vi "Spin Coat LbL Krizak SMS.vi"() -> ()   [LabVIEW 2018]
uses:
  <vilib>/ErrorRing/Error Ring.xnode
panel:
  in  "Units in 5":string(combo)="mh"
  in  "Set rate in 5":dbl=400.0
  in  "dia (mm) in 5":dbl=24.0 min=0.1 max=50.0 step=0.1
  in  "Units in 4":string(combo)="mh"
  in  "Set rate in 4":dbl=400.0
  in  "dia (mm) in 4":dbl=24.0 min=0.1 max=50.0 step=0.1
  in  "Units in 3":string(combo)="mh"
  in  "Set rate in 3":dbl=400.0
  in  "dia (mm) in 3":dbl=33.0 min=0.1 max=50.0 step=0.1
  in  "Units in 2":string(combo)="mh"
  in  "Set rate in 2":dbl=400.0
  in  "dia (mm) in 2":dbl=24.0 min=0.1 max=50.0 step=0.1
  out "Invalid Recipient":string
  in  "SMS Updates":bool=TRUE
  in  "Carrier":string(combo)="@tmomail.net"
  in  "Phone number":string="2816302191"
  out "Complete Indicator":bool caption="Start Button"
  in  "Activate Pump 5":bool
  out "Stopped 5":bool
  in  "Address in 5":string(combo)="0"
  in  "Target Vol (mL) 5":dbl=0.9
  out "Dispensed (mL) 5":dbl
  out "Success 5":bool
  out "Spin Coater":bool
  out "Pumps":bool
  out "Stopped 4":bool
  in  "Address in 4":string(combo)="3"
  in  "Target Vol (mL) 4":dbl=0.9
  out "Dispensed (mL) 4":dbl
  out "Success 4":bool
  out "Stopped 3":bool
  in  "Address in 3":string(combo)="4"
  in  "Target Vol (mL) 3":dbl=0.9
  out "Dispensed (mL) 3":dbl
  out "Success 3":bool
  out "Stopped 2":bool
  in  "Address in 2":string(combo)="1"
  in  "Target Vol (mL) 2":dbl=0.9
  out "Dispensed (mL) 2":dbl
  out "Success 2":bool
  out "Stopped 1":bool
  out "Pumps Reads":string
  out "Pump Commands":string
  out "Pump Reads Length":string
  in  "Address in 1":string(combo)="2"
  in  "Target Vol (mL) 1":dbl=0.9
  in  "Units in":string(combo)="mh"
  in  "Direction in":bool=TRUE
  in  "Set rate in":dbl=400.0
  in  "dia (mm) in":dbl=24.0 min=0.1 max=50.0 step=0.1
  in  "Pumps Serial Port":refnum<visa-resource-name>="COM1"
  out "Pump Operating":i32
  out "Layer #":i32=1
  out "String  After Match":string
  out "String  Before Match":string
  out "String  Match":string
  out "Spin Coater Stopped":bool
  in  "VISA resource name":refnum<visa-resource-name>="COM4" caption="Spin Coater Serial Port"
  out "Match 3":u8
  out "Match 2":u8
  out "Match 4":u8
  out "Match 5":u8
  out "Match 1":u8
  out "Match #":i32
  out "Spin Coater Reads":string
  out "error out":errorcluster
  in  "Stop All Button":bool caption="Start Button"
  out "Dispensed (mL) 1":dbl
  out "Success 1":bool
  in  "Number of Layers":i32=30
  # "Warning: This program must be started prior to starting the spin coater"
  # "Set pump Baud rate to 19200"
  # "Note: Spin Coater must be programmed independently for the correct number of cycles at a proper spin speed."
  # "Pump 1"
  # "Pump 2"
  # "Pump 5"
  # "Pump 3"
  # "Pump 4"
  # "Monomer 1"
  # "Rinse"
  # "Monomer 2"
  # "Rinse"
  # "Graphene"
  # "Diagnostics Panel"
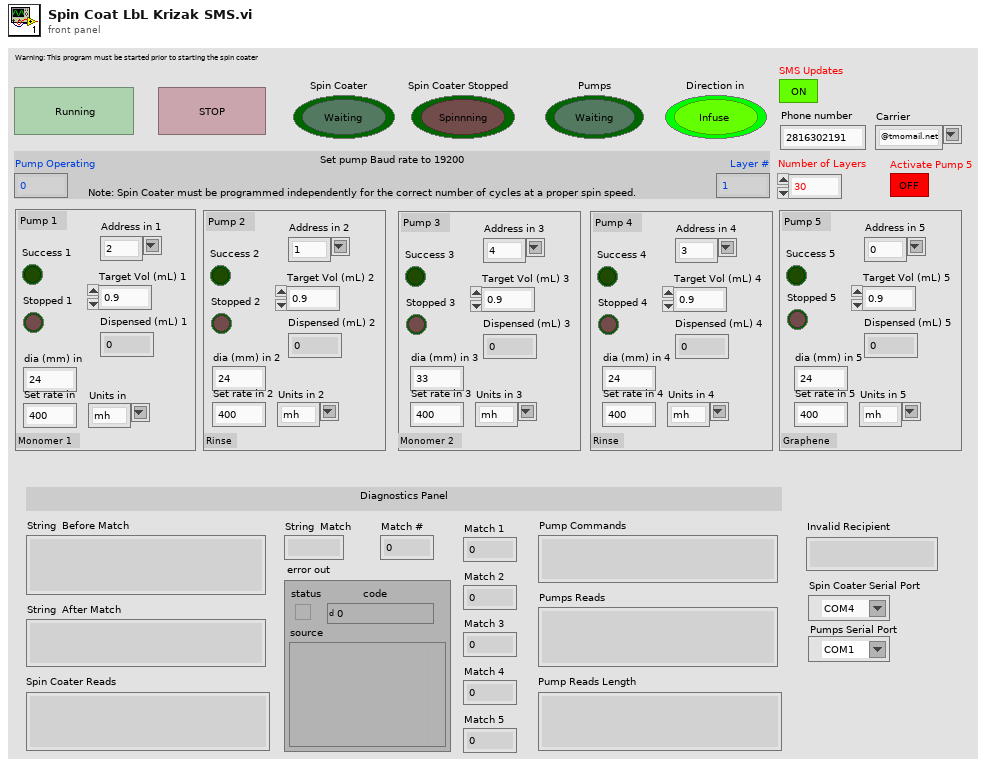
[diagram p1: front panel]
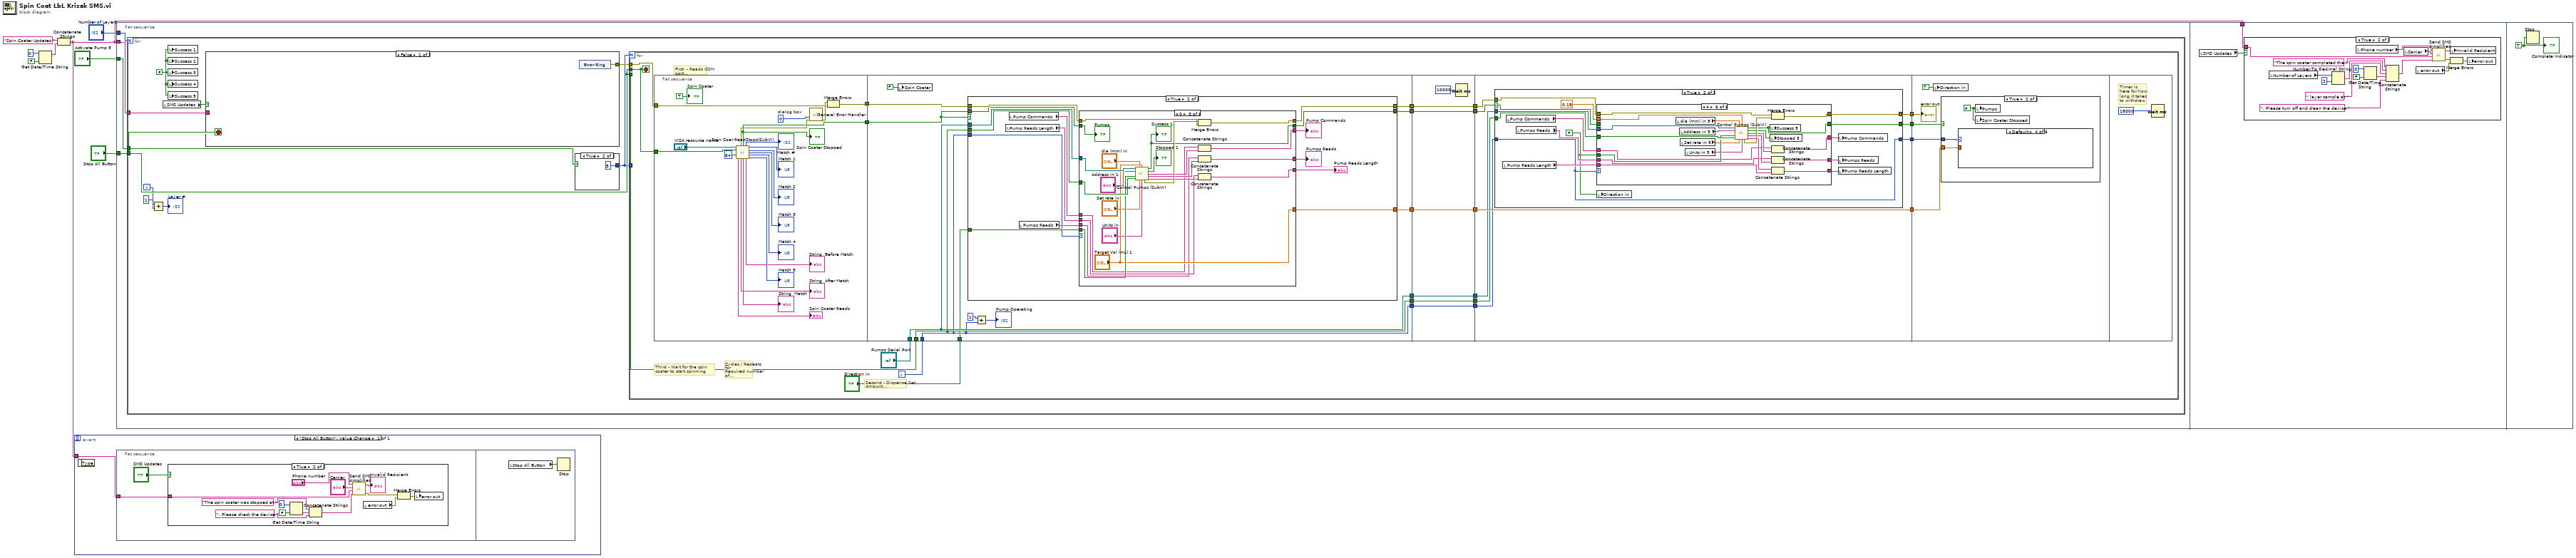
[diagram p0: block diagram]
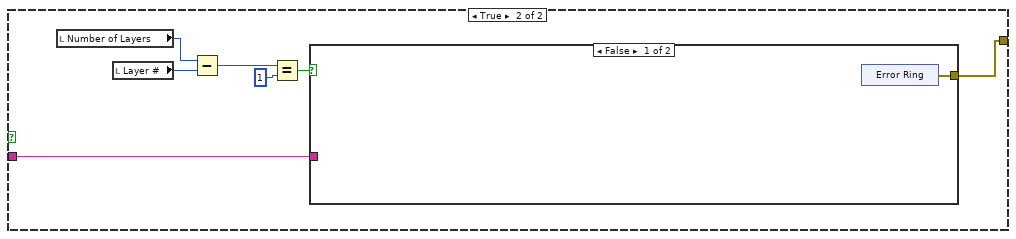
[diagram p2: hidden frame]
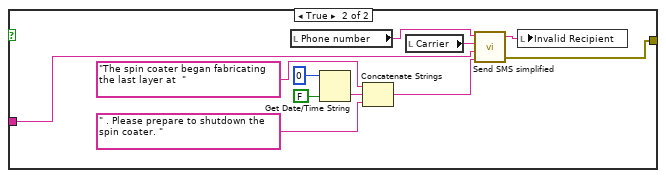
[diagram p3: hidden frame]
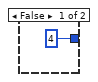
[diagram p4: hidden frame]
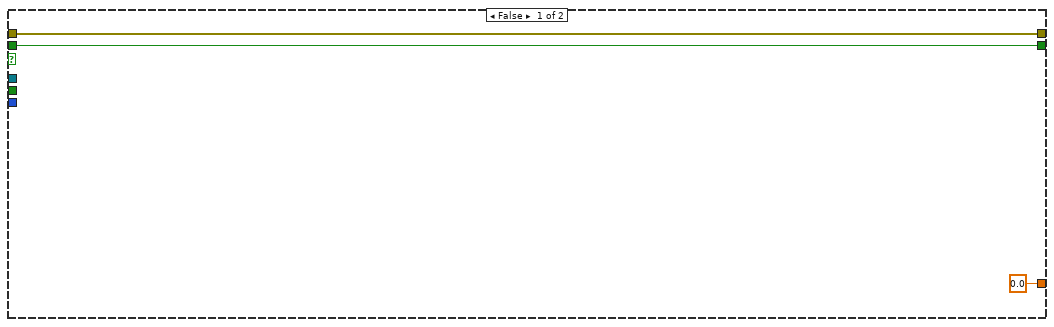
[diagram p5: hidden frame]
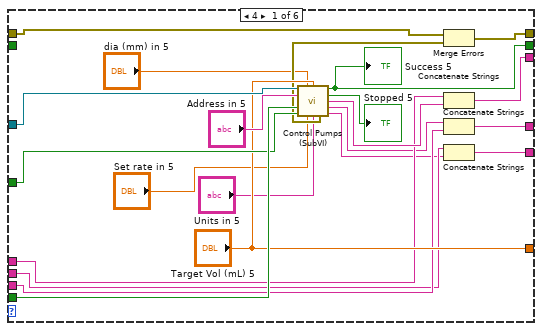
[diagram p6: hidden frame]
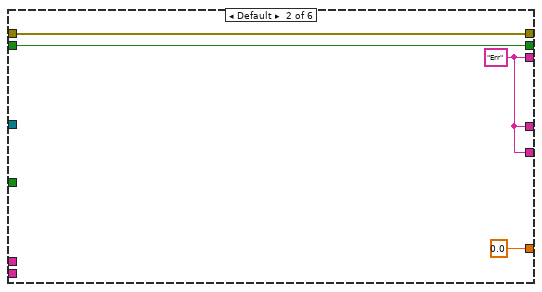
[diagram p7: hidden frame]
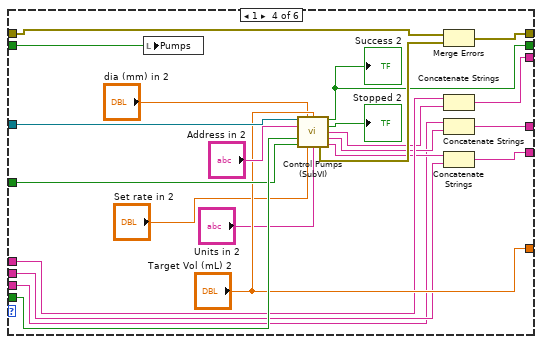
[diagram p8: hidden frame]
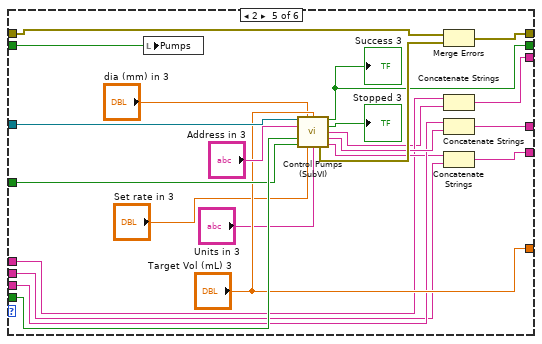
[diagram p9: hidden frame]
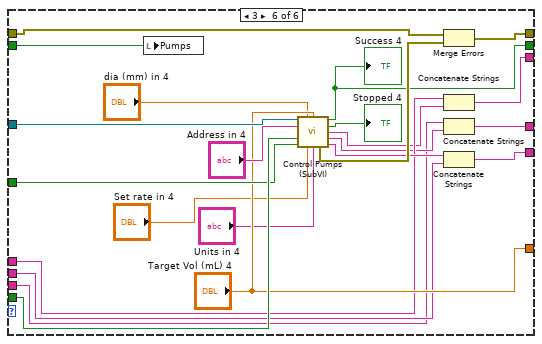
[diagram p10: hidden frame]
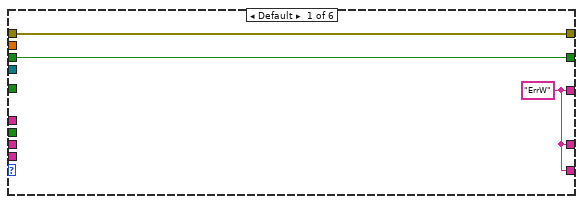
[diagram p12: hidden frame]
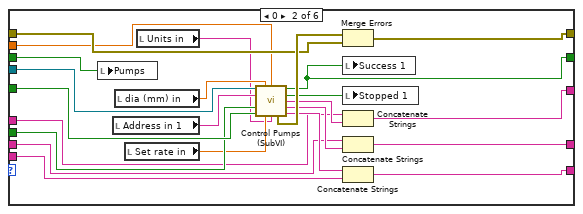
[diagram p13: hidden frame]
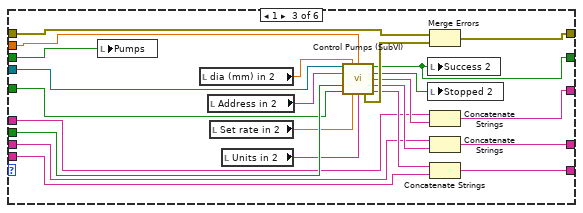
[diagram p14: hidden frame]
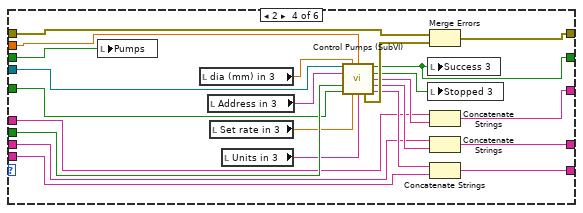
[diagram p15: hidden frame]
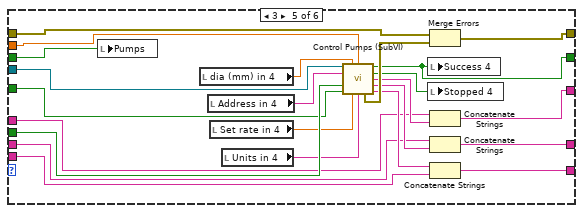
[diagram p16: hidden frame]
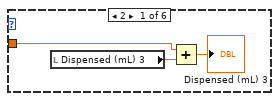
[diagram p18: hidden frame]
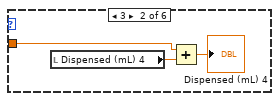
[diagram p19: hidden frame]
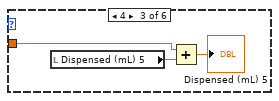
[diagram p20: hidden frame]
diagram:
  n1 = Get Date/Time String(date format (0)=i8 0 ("Number of pumps"), want seconds? (F)=FALSE) -> (date string=w2:string)  [unwired: 1 in, 1 out]
  n2 = Concatenate Strings("Spin Coater Updates ", w2) -> (w1:string)
  n3 = event shown="[0] \"Stop All Button\": Value Change" {
    selector: _ -> [_]
    dyn-events: _ -> [_]
    timeout: _ -> [_]
    tunnel: w1 -> [w9]
    event "Stop All Button": Value Change {
      n4 = event-data() -> ()  [unwired: 1 in, 1 out]
      n5 = flat-sequence {
        tunnel: w9 -> [w10]
        frame #0 {
          n6 = case shown="True" "SMS Updates" {
            tunnel: w10 -> [_ w23]
            frame False {
              n7 = xnode "Error Ring"() -> ()  [unwired: 1 out]
            }
            frame True {
              n8 = Get Date/Time String(date format (0)=i8 0 ("Number of pumps"), want seconds? (F)=FALSE) -> (time string=w19:string)  [unwired: 1 in, 1 out]
              n9 = Concatenate Strings("The spin coater was stopped at ", w19, ". Please check the device.") -> (w18:string)
              n10 = call "Send SMS simplified.vi"("Message"=w18, "Subject"=w23, "Carrier"="Carrier", "Phone number"="Phone number") -> ("Error Out"=w14:errorcluster, "Invalid Recipients"=→"Invalid Recipient":string)  [unwired: 1 in]
              n11 = local read "error out"() -> (w15:errorcluster)
              n12 = Merge Errors(w14, w15) -> (w13:errorcluster)
              n13 = local write "error out"(w13) -> ()
            }
          }
        }
        frame #1 {
          n14 = local read "Stop All Button"() -> (w26:bool)
          n15 = Stop(stop? (T)=w26) -> ()
        }
      }
    }
  }
  n16 = flat-sequence {
    tunnel: "Stop All Button" -> [w30]
    tunnel: "Activate Pump 5" -> [w29]
    tunnel: "Number of Layers" -> [w28]
    tunnel: w1 -> [w27]
    tunnel: w1 -> [w432]
    frame #0 {
      n17 = for {
        N: w28 -> [_]
        tunnel: w30 -> [w40]
        tunnel: w29 -> [w39]
        tunnel: w27 -> [w32]
        i -> [w37]
        stop <- w40 stop-if-true
        w34 = FALSE
        n18 = Add(x=1, y=w37) -> (x+y=→"Layer #":i32)
        n19 = local read "SMS Updates"() -> (w33:bool)
        n20 = local write "Success 1"(w34) -> ()
        n21 = local write "Success 2"(w34) -> ()
        n22 = local write "Success 3"(w34) -> ()
        n23 = local write "Success 4"(w34) -> ()
        n24 = local write "Success 5"(w34) -> ()
        n25 = case shown="False" w33 {
          tunnel: w32 -> [_ w44]
          tunnel: [w41 w43] -> w31
          frame False {
            n26 = xnode "Error Ring"() -> ("error out"=w41:errorcluster)
          }
          frame True {
            n27 = local read "Number of Layers"() -> (w49:i32)
            n28 = local read "Layer #"() -> (w48:i32)
            n29 = Subtract(x=w49, y=w48) -> (x-y=w46:i32)
            n30 = Equal?(x=w46, y=1) -> (x = y?=w47:bool)
            n31 = case shown="False" w47 {
              tunnel: w44 -> [_ w62]
              tunnel: [w50 w58] -> w43
              frame False {
                n32 = xnode "Error Ring"() -> ("error out"=w50:errorcluster)
              }
              frame True {
                n33 = local read "Phone number"() -> (w61:string)
                n34 = Get Date/Time String(date format (0)=i8 0 ("Number of pumps"), want seconds? (F)=FALSE) -> (time string=w55:string)  [unwired: 1 in, 1 out]
                n35 = Concatenate Strings("The spin coater began fabricating the last layer at  ", w55, " . Please prepare to shutdown the spin coater. ") -> (w53:string)
                n36 = local read "Carrier"() -> (w60:string)
                n37 = call "Send SMS simplified.vi"("Message"=w53, "Subject"=w62, "Carrier"=w60, "Phone number"=w61) -> ("Error Out"=w58:errorcluster, "Invalid Recipients"=w59:string)  [unwired: 1 in]
                n38 = local write "Invalid Recipient"(w59) -> ()
              }
            }
          }
        }
        n39 = case shown="True" w39 {
          tunnel: [4 ("Number of pumps") 5 ("Number of pumps")] -> w35
          frame False {
          }
          frame True {
          }
        }
        n40 = for {
          N: w35 -> [_]
          tunnel: w40 -> [w88]
          tunnel: w40 -> [w85]
          tunnel: w35 -> [_]
          tunnel: w31 -> [w65]
          i -> [w66]
          stop <- w88 stop-if-true
          # "Cycles / Repeats for \nRequired number of \nmonomers and\nlayers"
          # "Second - Dispense Set Amount\nfrom a given pump"
          # "Third - Wait for the spin \ncoater to start spinning"
          # "First  - Reads COM port\n   until spin coater stops"
          n41 = flat-sequence {
            tunnel: [w90] -> w87
            tunnel: [w105] -> w86
            tunnel: w88 -> [w107]
            tunnel: w65 -> [w89]
            tunnel: w87 -> [w120]
            tunnel: w86 -> [w115]
            tunnel: w66 -> [w110]
            tunnel: w85 -> [w112]
            tunnel: "Pumps Serial Port" -> [w114]
            tunnel: "Direction in" -> [w113]
            tunnel: [w119] -> w78
            tunnel: [w118] -> w76
            tunnel: [w110] -> w74
            tunnel: [w117] -> w72
            tunnel: [w114] -> w70
            tunnel: [w112] -> w68
            tunnel: w78 -> [w263]
            tunnel: [w263] -> w77
            tunnel: w76 -> [w262]
            tunnel: [w262] -> w75
            tunnel: w74 -> [w261]
            tunnel: [w261] -> w73
            tunnel: w72 -> [w260]
            tunnel: [w260] -> w71
            tunnel: w70 -> [w259]
            tunnel: [w259] -> w69
            tunnel: w68 -> [w258]
            tunnel: [w258] -> w67
            tunnel: w77 -> [w271]
            tunnel: w75 -> [w267]
            tunnel: w73 -> [w265]
            tunnel: [w264] -> w83
            tunnel: w71 -> [w272]
            tunnel: [w272] -> w82
            tunnel: [w270] -> w81
            tunnel: w69 -> [w269]
            tunnel: w67 -> [w268]
            tunnel: [w266] -> w79
            tunnel: w83 -> [w412]
            tunnel: w82 -> [w410]
            tunnel: w81 -> [w408]
            tunnel: w79 -> [w411]
            frame #0 {
              w92 = 0  # dialog box
              n42 = call "Spin Coar ReadStops(SubVI).vi"("VISA Refnum in"="VISA resource name", "stop"=w107, "bytes to read"=u32 64) -> ("error out"=w93:errorcluster, "Boolean"=w105:bool, "Match Number"=→"Match #":i32, "Match 1"=→"Match 1":u8, "Match 2"=→"Match 2":u8, "Match 3"=→"Match 3":u8, "Match 4"=→"Match 4":u8, "read string"=→"Spin Coater Reads":string, "String After Match"=→"String  After Match":string, "String Match"=→"String  Match":string, "String Before Match"=→"String  Before Match":string, "Match 5"=→"Match 5":u8)  [unwired: 1 in]
              "Spin Coater Stopped" <- w105
              n43 = call <vilib>:"General Error Handler.vi"("type of dialog (OK msg:1)"=w92, "error in (no error)"=w93) -> ("error out"=w91:errorcluster)  [unwired: 9 in, 4 out]
              n44 = Merge Errors(w91, w89) -> (w90:errorcluster)
              "Spin Coater" <- TRUE
            }
            frame #1 {
              n45 = local write "Spin Coater"(FALSE) -> ()
              n46 = case shown="True" w115 {
                tunnel: w120 -> [w123 w138]
                tunnel: w110 -> [_ w137]
                tunnel: w112 -> [_ w136]
                tunnel: w115 -> [w122 w130]
                tunnel: [w123 w135] -> w119
                tunnel: [w122 w134] -> w118
                tunnel: w114 -> [_ w133]
                tunnel: w113 -> [_ w132]
                tunnel: [0.0 w131] -> w117
                frame False {
                }
                frame True {
                  n47 = local read "Pump Reads Length"() -> (w126:string)
                  n48 = local read "Pump Commands"() -> (w125:string)
                  n49 = local read "Pumps Reads"() -> (w124:string)
                  n50 = case shown="0" w137 {
                    tunnel: w136 -> [w155 _ w185 w207 w227 w253]
                    tunnel: w130 -> [_ w161 w177 w200 w223 w246]
                    tunnel: w138 -> [w160 w164 w179 w205 w232 w252]
                    tunnel: [w159 w164 w187 w206 w231 w250] -> w135
                    tunnel: [w154 w161 w184 w201 w225 w249] -> w134
                    tunnel: w133 -> [w157 _ w183 w210 w230 w256]
                    tunnel: w132 -> [w156 _ w181 w208 w228 w254]
                    tunnel: ["Target Vol (mL) 5" 0.0 "Target Vol (mL) 1" "Target Vol (mL) 2" "Target Vol (mL) 3" "Target Vol (mL) 4"] -> w131
                    tunnel: [w143 w162 w173 w193 w221 w238] -> w129
                    tunnel: [w149 w162 w171 w191 w214 w240] -> w128
                    tunnel: [w142 w162 w175 w196 w218 w244] -> w127
                    tunnel: w126 -> [w146 _ w170 w198 w219 w243]
                    tunnel: w125 -> [w150 _ w168 w199 w216 w242]
                    tunnel: w124 -> [w147 _ w169 w194 w220 w237]
                    frame 4 {
                      n51 = call "Control Pumps (SubVI).vi"("VISA Refnum in"=w157, "Syringe Diameter (mm)"="dia (mm) in 5", "Target Vol (mL)"="Target Vol (mL) 5", "Address"="Address in 5", "Pumping Direction"=w156, "stop in"=w155, "Pumping Rate"="Set rate in 5", "Pumping Rate (unit)"="Units in 5") -> ("Success"=w154:bool, "Pump Stopped"=→"Stopped 5":bool, "concatenated string (Commands In)"=w151:string, "read buffer"=w148:string, "error out"=w144:errorcluster, "return counts (Read Length)"=w145:string)  [unwired: 2 in]
                      "Success 5" <- w154
                      n52 = Merge Errors(w160, w144) -> (w159:errorcluster)
                      n53 = Concatenate Strings(w150, w151) -> (w149:string)
                      n54 = Concatenate Strings(w148, w147) -> (w143:string)
                      n55 = Concatenate Strings(w146, w145) -> (w142:string)
                    }
                    frame Default {
                      w162 = "Err"
                    }
                    frame 0 {
                      n56 = call "Control Pumps (SubVI).vi"("VISA Refnum in"=w183, "Syringe Diameter (mm)"="dia (mm) in", "Target Vol (mL)"="Target Vol (mL) 1", "Address"="Address in 1", "Pumping Direction"=w181, "stop in"=w185, "Pumping Rate"="Set rate in", "Pumping Rate (unit)"="Units in") -> ("Success"=w184:bool, "Pump Stopped"=→"Stopped 1":bool, "concatenated string (Commands In)"=w172:string, "read buffer"=w174:string, "error out"=w186:errorcluster, "return counts (Read Length)"=w176:string)  [unwired: 2 in]
                      "Success 1" <- w184
                      n57 = Merge Errors(w186, w179) -> (w187:errorcluster)
                      n58 = Concatenate Strings(w168, w172) -> (w171:string)
                      n59 = Concatenate Strings(w169, w174) -> (w173:string)
                      n60 = Concatenate Strings(w170, w176) -> (w175:string)
                      "Pumps" <- w177
                    }
                    frame 1 {
                      n61 = local write "Pumps"(w200) -> ()
                      n62 = call "Control Pumps (SubVI).vi"("VISA Refnum in"=w210, "Syringe Diameter (mm)"="dia (mm) in 2", "Target Vol (mL)"="Target Vol (mL) 2", "Address"="Address in 2", "Pumping Direction"=w208, "stop in"=w207, "Pumping Rate"="Set rate in 2", "Pumping Rate (unit)"="Units in 2") -> ("Success"=w201:bool, "Pump Stopped"=→"Stopped 2":bool, "concatenated string (Commands In)"=w192:string, "read buffer"=w195:string, "error out"=w204:errorcluster, "return counts (Read Length)"=w197:string)  [unwired: 2 in]
                      "Success 2" <- w201
                      n63 = Merge Errors(w205, w204) -> (w206:errorcluster)
                      n64 = Concatenate Strings(w199, w192) -> (w191:string)
                      n65 = Concatenate Strings(w194, w195) -> (w193:string)
                      n66 = Concatenate Strings(w197, w198) -> (w196:string)
                    }
                    frame 2 {
                      n67 = local write "Pumps"(w223) -> ()
                      n68 = call "Control Pumps (SubVI).vi"("VISA Refnum in"=w230, "Syringe Diameter (mm)"="dia (mm) in 3", "Target Vol (mL)"="Target Vol (mL) 3", "Address"="Address in 3", "Pumping Direction"=w228, "stop in"=w227, "Pumping Rate"="Set rate in 3", "Pumping Rate (unit)"="Units in 3") -> ("Success"=w225:bool, "Pump Stopped"=→"Stopped 3":bool, "concatenated string (Commands In)"=w215:string, "read buffer"=w222:string, "error out"=w233:errorcluster, "return counts (Read Length)"=w217:string)  [unwired: 2 in]
                      "Success 3" <- w225
                      n69 = Merge Errors(w232, w233) -> (w231:errorcluster)
                      n70 = Concatenate Strings(w216, w215) -> (w214:string)
                      n71 = Concatenate Strings(w220, w222) -> (w221:string)
                      n72 = Concatenate Strings(w217, w219) -> (w218:string)
                    }
                    frame 3 {
                      n73 = local write "Pumps"(w246) -> ()
                      n74 = call "Control Pumps (SubVI).vi"("VISA Refnum in"=w256, "Syringe Diameter (mm)"="dia (mm) in 4", "Target Vol (mL)"="Target Vol (mL) 4", "Address"="Address in 4", "Pumping Direction"=w254, "stop in"=w253, "Pumping Rate"="Set rate in 4", "Pumping Rate (unit)"="Units in 4") -> ("Success"=w249:bool, "Pump Stopped"=→"Stopped 4":bool, "concatenated string (Commands In)"=w241:string, "read buffer"=w239:string, "error out"=w251:errorcluster, "return counts (Read Length)"=w245:string)  [unwired: 2 in]
                      "Success 4" <- w249
                      n75 = Merge Errors(w252, w251) -> (w250:errorcluster)
                      n76 = Concatenate Strings(w242, w241) -> (w240:string)
                      n77 = Concatenate Strings(w237, w239) -> (w238:string)
                      n78 = Concatenate Strings(w245, w243) -> (w244:string)
                    }
                  }
                  "Pump Reads Length" <- w127
                  "Pump Commands" <- w128
                  "Pumps Reads" <- w129
                }
              }
              n79 = Add(x=1, y=w110) -> (x+y=→"Pump Operating":i32)
            }
            frame #2 {
              n80 = Wait (ms)(milliseconds to wait=u32 10000) -> ()  [unwired: 1 out]
            }
            frame #3 {
              n81 = case shown="True" w267 {
                selector: w267 -> [w273 w277]
                tunnel: w271 -> [w275 w290]
                tunnel: w265 -> [w274 w278]
                tunnel: w268 -> [_ w289]
                tunnel: [w275 w288] -> w270
                tunnel: [w273 w287] -> w266
                tunnel: w269 -> [_ w286]
                tunnel: [w274 w278] -> w264
                frame False {
                }
                frame True {
                  w276 = FALSE
                  n82 = local read "Pump Reads Length"() -> (w281:string)
                  n83 = local read "Pump Commands"() -> (w279:string)
                  n84 = local read "Pumps Reads"() -> (w280:string)
                  n85 = case shown="4" w278 {
                    tunnel: w289 -> [_ w314 w337 w357 w383 w398]
                    tunnel: w277 -> [w291 w306 w333 w356 w379 _]
                    tunnel: w290 -> [w293 w311 w335 w361 w382 w389]
                    tunnel: [w293 w316 w336 w360 w380 w390] -> w288
                    tunnel: [w291 w308 w329 w353 w375 w391] -> w287
                    tunnel: w286 -> [_ w313 w339 w359 w385 w395]
                    tunnel: w276 -> [_ w312 w338 w358 w384 w397]
                    tunnel: [w292 w302 w324 w347 w371 w403] -> w283
                    tunnel: [w292 w300 w322 w345 w367 w392] -> w284
                    tunnel: [w292 w304 w327 w350 w373 w404] -> w282
                    tunnel: 0.15 -> [_ w310 w332 w355 w378 w399]
                    tunnel: w281 -> [_ w299 w326 w349 w372 w405]
                    tunnel: w280 -> [_ w298 w321 w344 w369 w401]
                    tunnel: w279 -> [_ w297 w320 w343 w366 w394]
                    frame Default {
                      w292 = "ErrW"
                    }
                    frame 0 {
                      n86 = local write "Pumps"(w306) -> ()
                      n87 = local read "Address in 1"() -> (w309:string)
                      n88 = local read "dia (mm) in"() -> (w296:dbl)
                      n89 = local read "Set rate in"() -> (w295:dbl)
                      n90 = local read "Units in"() -> (w294:string)
                      n91 = call "Control Pumps (SubVI).vi"("VISA Refnum in"=w313, "Syringe Diameter (mm)"=w296, "Target Vol (mL)"=w310, "Address"=w309, "Pumping Direction"=w312, "stop in"=w314, "Pumping Rate"=w295, "Pumping Rate (unit)"=w294) -> ("Success"=w308:bool, "Pump Stopped"=w307:bool, "concatenated string (Commands In)"=w301:string, "read buffer"=w303:string, "error out"=w315:errorcluster, "return counts (Read Length)"=w305:string)  [unwired: 2 in]
                      n92 = Merge Errors(w315, w311) -> (w316:errorcluster)
                      n93 = local write "Success 1"(w308) -> ()
                      n94 = local write "Stopped 1"(w307) -> ()
                      n95 = Concatenate Strings(w297, w301) -> (w300:string)
                      n96 = Concatenate Strings(w298, w303) -> (w302:string)
                      n97 = Concatenate Strings(w305, w299) -> (w304:string)
                    }
                    frame 1 {
                      n98 = local write "Pumps"(w333) -> ()
                      n99 = local read "dia (mm) in 2"() -> (w319:dbl)
                      n100 = local read "Address in 2"() -> (w331:string)
                      n101 = local read "Set rate in 2"() -> (w318:dbl)
                      n102 = local read "Units in 2"() -> (w317:string)
                      n103 = call "Control Pumps (SubVI).vi"("VISA Refnum in"=w339, "Syringe Diameter (mm)"=w319, "Target Vol (mL)"=w332, "Address"=w331, "Pumping Direction"=w338, "stop in"=w337, "Pumping Rate"=w318, "Pumping Rate (unit)"=w317) -> ("Success"=w329:bool, "Pump Stopped"=w330:bool, "concatenated string (Commands In)"=w323:string, "read buffer"=w325:string, "error out"=w334:errorcluster, "return counts (Read Length)"=w328:string)  [unwired: 2 in]
                      n104 = local write "Success 2"(w329) -> ()
                      n105 = local write "Stopped 2"(w330) -> ()
                      n106 = Merge Errors(w335, w334) -> (w336:errorcluster)
                      n107 = Concatenate Strings(w320, w323) -> (w322:string)
                      n108 = Concatenate Strings(w321, w325) -> (w324:string)
                      n109 = Concatenate Strings(w328, w326) -> (w327:string)
                    }
                    frame 2 {
                      n110 = local write "Pumps"(w356) -> ()
                      n111 = local read "dia (mm) in 3"() -> (w340:dbl)
                      n112 = local read "Address in 3"() -> (w354:string)
                      n113 = local read "Set rate in 3"() -> (w341:dbl)
                      n114 = local read "Units in 3"() -> (w342:string)
                      n115 = call "Control Pumps (SubVI).vi"("VISA Refnum in"=w359, "Syringe Diameter (mm)"=w340, "Target Vol (mL)"=w355, "Address"=w354, "Pumping Direction"=w358, "stop in"=w357, "Pumping Rate"=w341, "Pumping Rate (unit)"=w342) -> ("Success"=w353:bool, "Pump Stopped"=w352:bool, "concatenated string (Commands In)"=w346:string, "read buffer"=w348:string, "error out"=w362:errorcluster, "return counts (Read Length)"=w351:string)  [unwired: 2 in]
                      n116 = local write "Success 3"(w353) -> ()
                      n117 = local write "Stopped 3"(w352) -> ()
                      n118 = Merge Errors(w361, w362) -> (w360:errorcluster)
                      n119 = Concatenate Strings(w343, w346) -> (w345:string)
                      n120 = Concatenate Strings(w344, w348) -> (w347:string)
                      n121 = Concatenate Strings(w351, w349) -> (w350:string)
                    }
                    frame 3 {
                      n122 = local write "Pumps"(w379) -> ()
                      n123 = local read "dia (mm) in 4"() -> (w363:dbl)
                      n124 = local read "Address in 4"() -> (w377:string)
                      n125 = local read "Set rate in 4"() -> (w364:dbl)
                      n126 = local read "Units in 4"() -> (w365:string)
                      n127 = call "Control Pumps (SubVI).vi"("VISA Refnum in"=w385, "Syringe Diameter (mm)"=w363, "Target Vol (mL)"=w378, "Address"=w377, "Pumping Direction"=w384, "stop in"=w383, "Pumping Rate"=w364, "Pumping Rate (unit)"=w365) -> ("Success"=w375:bool, "Pump Stopped"=w376:bool, "concatenated string (Commands In)"=w368:string, "read buffer"=w370:string, "error out"=w381:errorcluster, "return counts (Read Length)"=w374:string)  [unwired: 2 in]
                      n128 = local write "Success 4"(w375) -> ()
                      n129 = local write "Stopped 4"(w376) -> ()
                      n130 = Merge Errors(w382, w381) -> (w380:errorcluster)
                      n131 = Concatenate Strings(w366, w368) -> (w367:string)
                      n132 = Concatenate Strings(w369, w370) -> (w371:string)
                      n133 = Concatenate Strings(w374, w372) -> (w373:string)
                    }
                    frame 4 {
                      n134 = local read "dia (mm) in 5"() -> (w388:dbl)
                      n135 = local read "Address in 5"() -> (w396:string)
                      n136 = local read "Set rate in 5"() -> (w387:dbl)
                      n137 = local read "Units in 5"() -> (w386:string)
                      n138 = call "Control Pumps (SubVI).vi"("VISA Refnum in"=w395, "Syringe Diameter (mm)"=w388, "Target Vol (mL)"=w399, "Address"=w396, "Pumping Direction"=w397, "stop in"=w398, "Pumping Rate"=w387, "Pumping Rate (unit)"=w386) -> ("Success"=w391:bool, "Pump Stopped"=w400:bool, "concatenated string (Commands In)"=w393:string, "read buffer"=w402:string, "error out"=w407:errorcluster, "return counts (Read Length)"=w406:string)  [unwired: 2 in]
                      n139 = local write "Success 5"(w391) -> ()
                      n140 = local write "Stopped 5"(w400) -> ()
                      n141 = Merge Errors(w389, w407) -> (w390:errorcluster)
                      n142 = Concatenate Strings(w394, w393) -> (w392:string)
                      n143 = Concatenate Strings(w401, w402) -> (w403:string)
                      n144 = Concatenate Strings(w406, w405) -> (w404:string)
                    }
                  }
                  n145 = local write "Direction in"(w276) -> ()
                  n146 = local write "Pump Commands"(w284) -> ()
                  n147 = local write "Pumps Reads"(w283) -> ()
                  n148 = local write "Pump Reads Length"(w282) -> ()
                }
              }
            }
            frame #4 {
              n149 = local write "Direction in"(TRUE) -> ()
              n150 = case shown="True" w411 {
                tunnel: w412 -> [_ w415]
                tunnel: w410 -> [_ w414]
                frame False {
                }
                frame True {
                  w413 = FALSE
                  n151 = case shown="Default" w415 {
                    tunnel: w414 -> [w417 w420 w422 _ w426 w428]
                    frame 2 {
                      n152 = local read "Dispensed (mL) 3"() -> (w418:dbl)
                      n153 = Add(x=w417, y=w418) -> (x+y=→"Dispensed (mL) 3":dbl)
                    }
                    frame 3 {
                      n154 = local read "Dispensed (mL) 4"() -> (w421:dbl)
                      n155 = Add(x=w420, y=w421) -> (x+y=→"Dispensed (mL) 4":dbl)
                    }
                    frame 4 {
                      n156 = local read "Dispensed (mL) 5"() -> (w424:dbl)
                      n157 = Add(x=w422, y=w424) -> (x+y=→"Dispensed (mL) 5":dbl)
                    }
                    frame Default {
                    }
                    frame 0 {
                      n158 = local read "Dispensed (mL) 1"() -> (w427:dbl)
                      n159 = Add(x=w426, y=w427) -> (x+y=→"Dispensed (mL) 1":dbl)
                    }
                    frame 1 {
                      n160 = local read "Dispensed (mL) 2"() -> (w430:dbl)
                      n161 = Add(x=w428, y=w430) -> (x+y=→"Dispensed (mL) 2":dbl)
                    }
                  }
                  n162 = local write "Pumps"(w413) -> ()
                  n163 = local write "Spin Coater Stopped"(w413) -> ()
                }
              }
              "error out" <- w408
            }
            frame #5 {
              # "Timer is here for how long it takes to withdraw"
              n164 = Wait (ms)(milliseconds to wait=u32 18000) -> ()  [unwired: 1 out]
            }
          }
        }
      }
    }
    frame #1 {
      n165 = local read "SMS Updates"() -> (w433:bool)
      n166 = case shown="True" w433 {
        tunnel: w432 -> [_ w439]
        frame False {
        }
        frame True {
          n167 = local read "Number of Layers"() -> (w445:i32)
          n168 = Number To Decimal String(number=w445, width (-)=i8 2 ("Number of pumps")) -> (decimal integer string=w443:string)
          n169 = local read "Phone number"() -> (w438:string)
          n170 = Get Date/Time String(date format (0)=i8 0 ("Number of pumps"), want seconds? (F)=FALSE) -> (time string=w441:string)  [unwired: 1 in, 1 out]
          n171 = Concatenate Strings("The spin coater completed the ", w443, " layer sample at ", w441, ". Please turn off and clean the device.") -> (w447:string)
          n172 = local read "Carrier"() -> (w446:string)
          n173 = local read "error out"() -> (w436:errorcluster)
          n174 = call "Send SMS simplified.vi"("Message"=w447, "Subject"=w439, "Carrier"=w446, "Phone number"=w438) -> ("Error Out"=w434:errorcluster, "Invalid Recipients"=w437:string)  [unwired: 1 in]
          n175 = local write "Invalid Recipient"(w437) -> ()
          n176 = Merge Errors(w434, w436) -> (w435:errorcluster)
          n177 = local write "error out"(w435) -> ()
        }
      }
    }
    frame #2 {
      w451 = TRUE
      n178 = Stop(stop? (T)=w451) -> ()
      "Complete Indicator" <- w451
    }
  }
